vi "Acquisition.vi"(11 "Acq Msg":T2) -> (4 "Display Stream":T1, 5 "Log Stream":T1, 6 "UI Msg":T2)   [LabVIEW 2019, in "Acquisition.lvlib"]
doc: "Message loop for handling messages pertaining to the acquisition of data from the hardware."
uses:
  Acquisition.lvlib
  <extravilib>/ChannelInstances/Messenger-t'Message Queue.lvlib-Message Cluster.ctl'/))Channel.ctl
  support/Message Queue/Message Cluster.ctl
  <extravilib>/ChannelInstances/Stream-var/)Channel.ctl
  HeatFlow/HeatFlow HW Tasks.ctl
  Acquisition State.ctl
  Settings/Settings.ctl
  Settings/Runtime Conf.ctl
  HeatFlow/HeatFlow HW Cfg.ctl
  HeatFlow/HeatFlow Acq Data.ctl
  <extravilib>/ChannelInstances/Stream-var/Write With Abort.vi
  <extravilib>/ChannelInstances/Stream-var/Endpoint.vi
  <extravilib>/ChannelInstances/Messenger-t'Message Queue.lvlib-Message Cluster.ctl'/Instantiate.vi
  <vilib>/Utility/error.llb/Error Cluster From Error Code.vi
  <extravilib>/ChannelInstances/Stream-var/)Channel.vi
  <resource>/ChannelSupport/_ChannelSupport/WaitIfNeeded.vi
  <vilib>/ErrorRing/Error Ring.xnode
  support/Message Queue/Message Queue.lvlib
  Settings/Settings.lvlib
  <extravilib>/ChannelInstances/Stream-var.lvlib
  <extravilib>/ChannelInstances/Messenger-t'Message Queue.lvlib-Message Cluster.ctl'.lvlib
panel:
  in  "Wart zwrotna":dbl
  out "Time":dbl
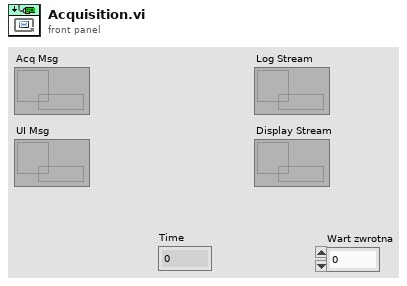
[diagram p1: front panel]
types:
  T1 = typedef "Stream-var.lvlib/)Channel.ctl" = refnum<queue>
  T2 = typedef "Messenger-t'Message Queue.lvlib-Message Cluster.ctl'.lvlib/))Channel.ctl" = refnum<queue>
  T3 = typedef "Acquisition.lvlib/HeatFlow HW Cfg.ctl" = cluster{"Heater Temp":cluster{"On":bool, "Min Val":dbl, "Max Val":dbl, "Units":string}, "LakeShore Temp":cluster{"On":bool, "Min Val":dbl, "Max Val":dbl, "Units":string}, "Heater Ctrl":cluster{"On":bool, "Min Val":dbl, "Max Val":dbl}, "TEG Load dU":cluster{"On":bool, "Min Val":dbl, "Max Val":dbl}, "Heater dU":cluster{"On":bool, "Min Val":dbl, "Max Val":dbl}, "I Res dU":cluster{"On":bool, "Min Val":dbl, "Max Val":dbl}, "Is Conf Set Up":bool}
  T4 = typedef "Settings.lvlib/Settings.ctl" = cluster{"Runtime":T5, "Cfg Files Dir":path, "Cfg File":path}
  T5 = typedef "Settings.lvlib/Runtime Conf.ctl" = cluster{"Time Interval, s":dbl, "Time Resolution, ms":u32, "Hot Side MOS, V":dbl, "Cold Side MOS, V":dbl}
  T6 = typedef "Acquisition.lvlib/Acquisition State.ctl" = enum16{"Idle", "Acquiring"}
  T7 = typedef "Acquisition.lvlib/HeatFlow HW Tasks.ctl" = cluster{"Heater Temp Task":refnum<k21>, "Heater Ctrl Task":refnum<k21>, "TEG Load dU Task":refnum<k21>, "Heater dU Task":refnum<k21>, "I Res dU Task":refnum<k21>, "LakeShore Temp":refnum<visa-resource-name>}
  T8 = typedef "Logging.lvlib/HeatFlow Res Cfg.ctl" = cluster{"Heater Temp":cluster{"On":bool, "Min Val":dbl, "Max Val":dbl, "Units":string}, "Tube Temp":cluster{"On":bool, "Min Val":dbl, "Max Val":dbl, "Units":string}, "Hot Heater Power":cluster{"On":bool, "Min Val":dbl, "Max Val":dbl, "Units":string}, "TEG Power":cluster{"On":bool, "Min Val":dbl, "Max Val":dbl, "Units":string}, "Details":bool, "Heater dU":cluster{"Min Val":dbl, "Max Val":dbl, "Units":string}, "I Res dU":cluster{"Min Val":dbl, "Max Val":dbl, "Units":string}}
  T9 = typedef "Acquisition.lvlib/HeatFlow Acq Data.ctl" = cluster{"Time Stamp":timestamp, "Time Delta":u32, "LakeShore_Temp":cluster{"Tube_T_1":dbl, "Tube_T_2":dbl, "Tube_T_3":dbl, "Tube_T_4":dbl, "Tube_T_5":dbl, "Tube_T_6":dbl, "Tube_T_7":dbl, "Tube_T_8":dbl}, "Heaters":cluster{"I_Res_dU":dbl, "Heater_dU":dbl, "Hot_Side_I":dbl, "Hot_Side_P":dbl, "Cold_Ctrl_U":dbl, "Hot_Ctrl_U":dbl, "Hot_Side_T":dbl, "Cold_Side_T":dbl}, "TEG":cluster{"TEG_Load_dU":dbl, "TEG_Load_R":dbl, "TEG_Load_I":dbl, "TEG_Load_P":dbl, "TEG_eta":dbl, "TEG_dT":dbl, "TEG_U_open":dbl, "TEG_U_Test":dbl, "TEG_R_Test":dbl, "TEG_Rw":dbl}, "LastElement?":bool}
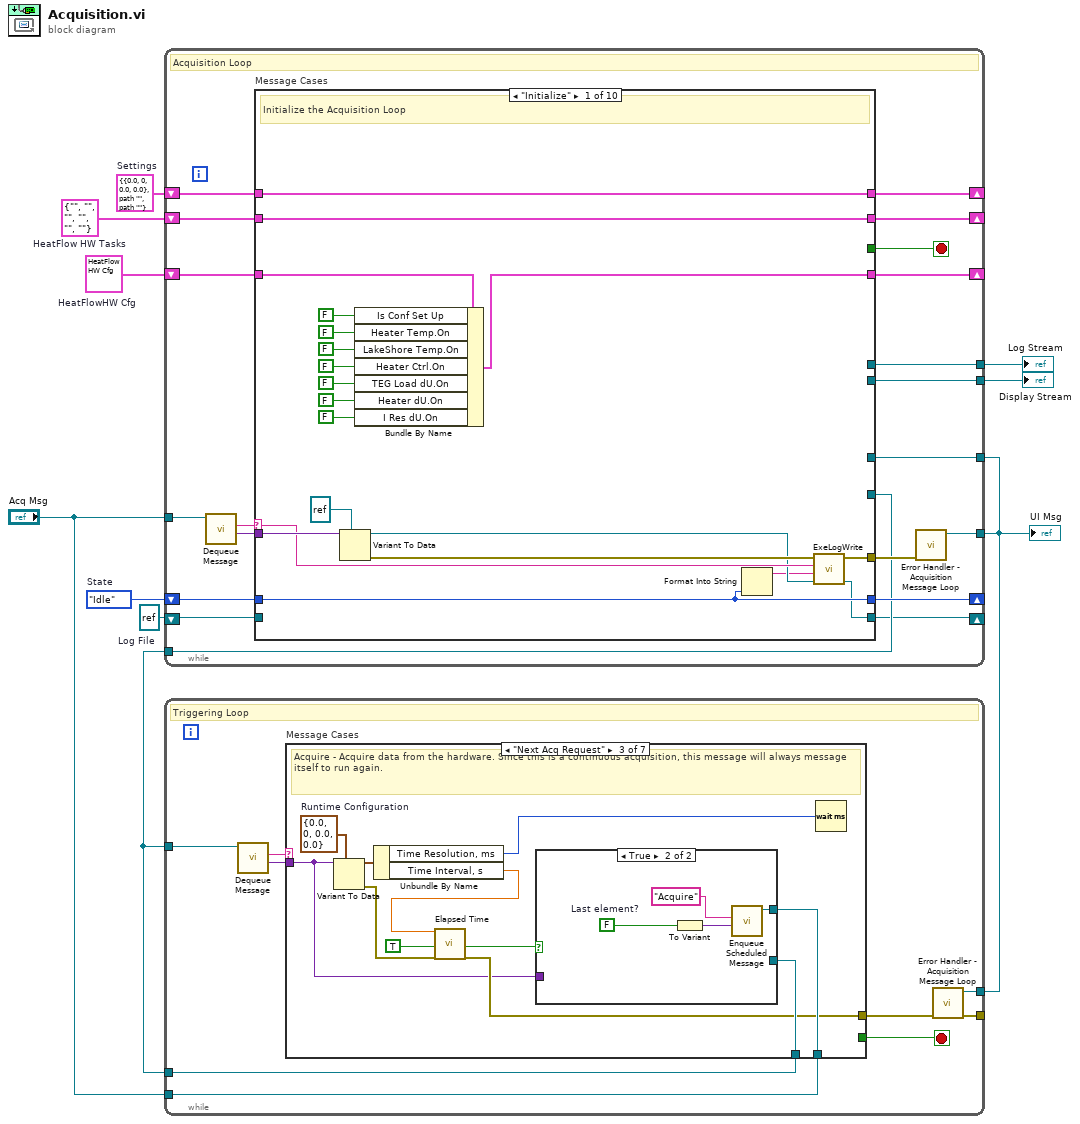
[diagram p0: block diagram]
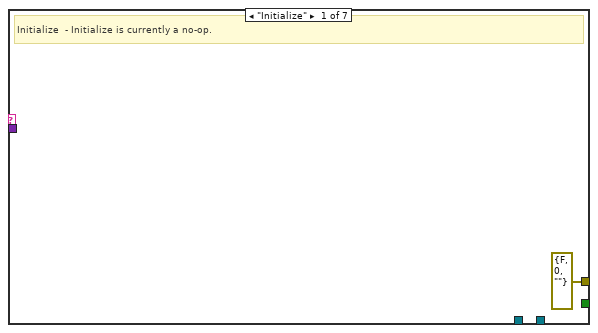
[diagram p2: hidden frame]
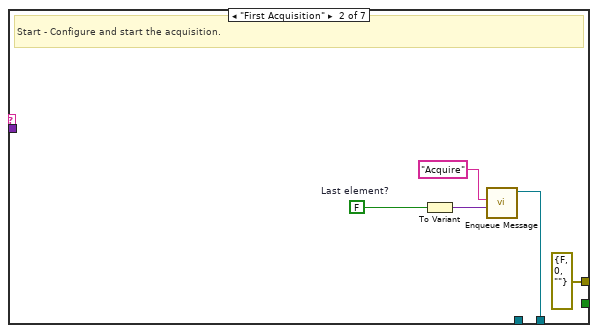
[diagram p3: hidden frame]
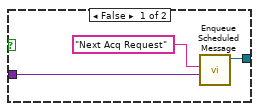
[diagram p4: hidden frame]
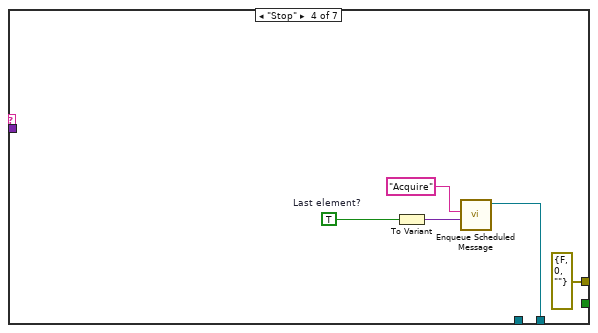
[diagram p5: hidden frame]
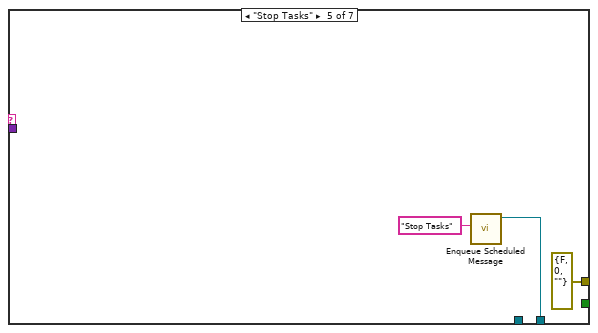
[diagram p6: hidden frame]
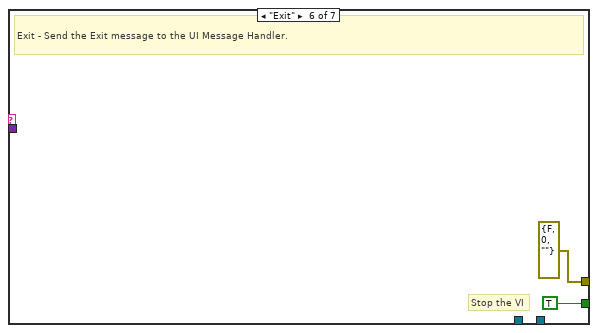
[diagram p7: hidden frame]
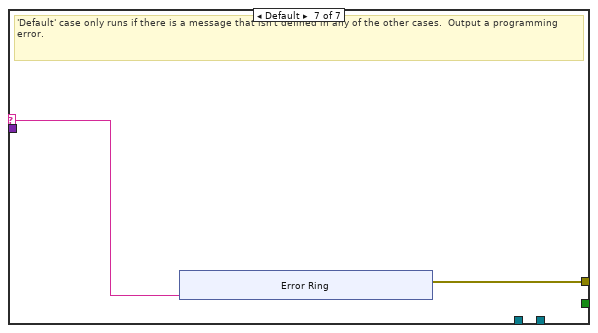
[diagram p8: hidden frame]
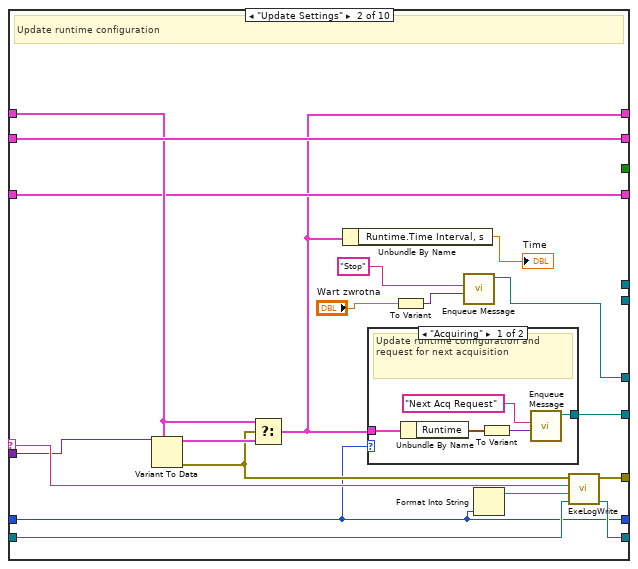
[diagram p9: hidden frame]
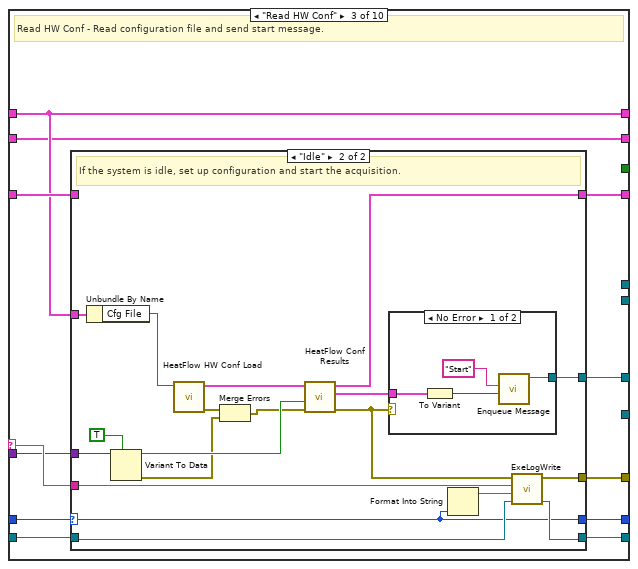
[diagram p11: hidden frame]
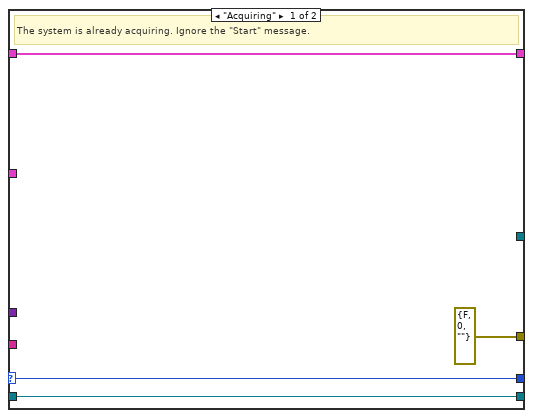
[diagram p12: hidden frame]
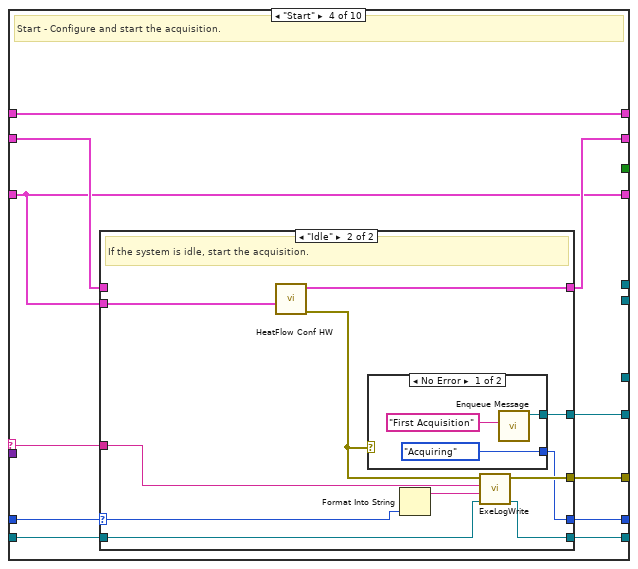
[diagram p14: hidden frame]
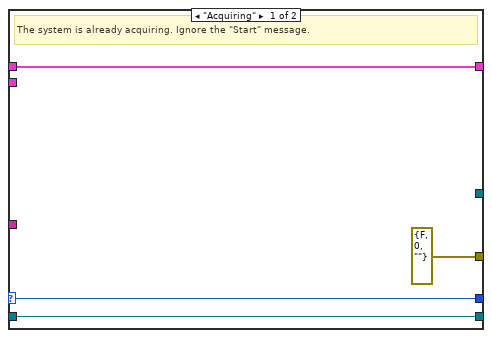
[diagram p15: hidden frame]
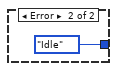
[diagram p16: hidden frame]
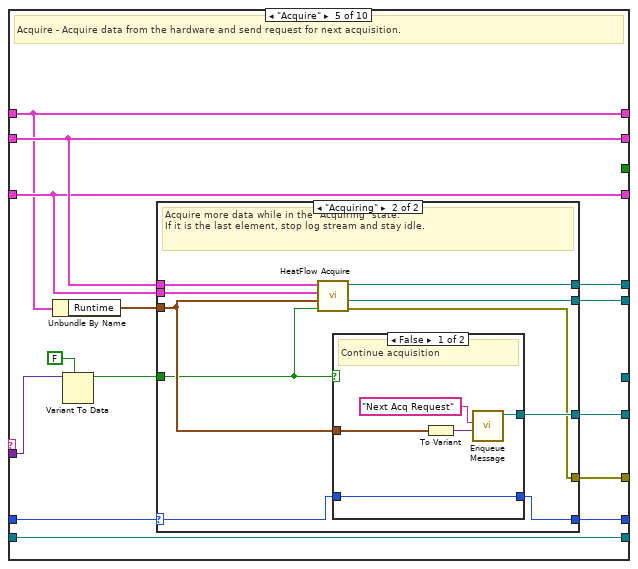
[diagram p17: hidden frame]
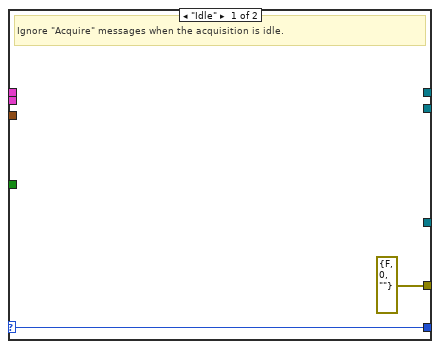
[diagram p18: hidden frame]
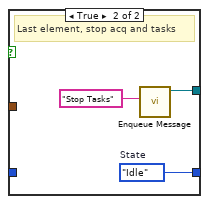
[diagram p19: hidden frame]
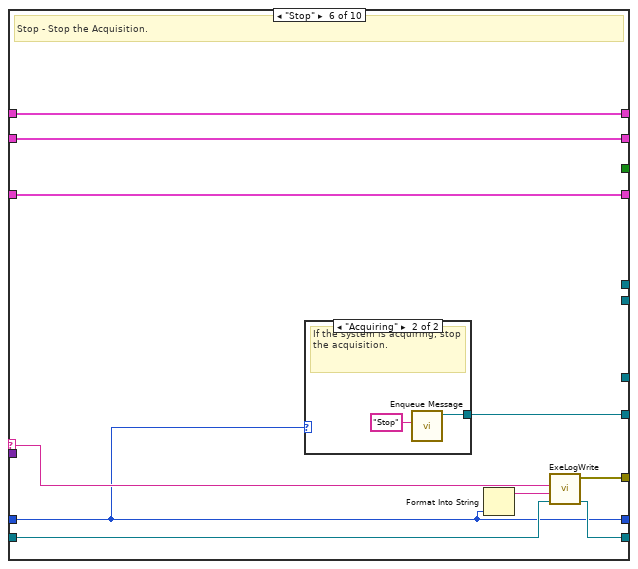
[diagram p20: hidden frame]
diagram:
  w1 = T3 {"Heater Temp"={"On"=FALSE, "Min Val"=0.0, "Max Val"=0.0, "Units"=""}, "LakeShore Temp"={"On"=FALSE, "Min Val"=0.0, "Max Val"=0.0, "Units"=""}, "Heater Ctrl"={"On"=FALSE, "Min Val"=0.0, "Max Val"=0.0}, "TEG Load dU"={"On"=FALSE, "Min Val"=0.0, "Max Val"=0.0}, "Heater dU"={"On"=FALSE, "Min Val"=0.0, "Max Val"=0.0}, "I Res dU"={"On"=FALSE, "Min Val"=0.0, "Max Val"=0.0}, "Is Conf Set Up"=FALSE}  # HeatFlowHW Cfg
  w4 = T4 {"Runtime"={"Time Interval, s"=0.0, "Time Resolution, ms"=0, "Hot Side MOS, V"=0.0, "Cold Side MOS, V"=0.0}, "Cfg Files Dir"=path "", "Cfg File"=path ""}  # Settings
  w5 = refnum<file> refnum  # Log File
  w7 = Acquisition_State."Idle"  # State
  w8 = T7 {"Heater Temp Task"="", "Heater Ctrl Task"="", "TEG Load dU Task"="", "Heater dU Task"="", "I Res dU Task"="", "LakeShore Temp"=""}  # HeatFlow HW Tasks
  n1 = while {
    shift-right: [w29] -> _
    shift-left: w8 -> [w30]
    shift-right: [w27] -> _
    shift-left: w7 -> [w28]
    shift-right: [w25] -> _
    shift-left: w4 -> [w26]
    tunnel: "Acq Msg" -> [w19]
    tunnel: [w21] -> w10
    tunnel: w10 -> [w20]
    tunnel: w6 -> [w18]
    shift-right: [w15] -> _
    shift-left: w5 -> [w16]
    shift-right: [w13] -> _
    shift-left: w1 -> [w14]
    tunnel: [w12] -> w3
    tunnel: [w11] -> w2
    stop <- w17 stop-if-true
    # "Acquisition Loop"
    n2 = call "Dequeue Message.vi"("channel"=w19) -> ("message data"=w23:variant, "message"=w24:string)  [unwired: 8 in, 1 out]
    n3 = case "Message Cases" shown="\"Initialize\"" w24 {
      selector: w24 -> [w45 w66 w81 w118 _ w183 w196 w213 w234 w245]
      tunnel: [w41 w65 w86 w124 w157 w181 w193 w214 w229 w246] -> w22
      tunnel: w30 -> [w50 w62 w76 w116 w152 w180 w192 w212 w241 w248]
      tunnel: [w50 w62 w76 w115 w152 w180 w192 w212 w241 w248] -> w29
      tunnel: w28 -> [w43 w57 w84 w122 w155 w178 w190 w207 w235 w247]
      tunnel: [w43 w57 w85 w123 w156 w178 w190 w207 w235 w247] -> w27
      tunnel: w26 -> [w49 w59 w78 w117 w149 w187 w200 w210 w240 w244]
      tunnel: [w49 w56 w78 w117 w149 w187 w200 w210 w240 w244] -> w25
      tunnel: w23 -> [w47 w63 w75 _ w147 _ _ _ _ _]
      tunnel: [_ w60 _ w121 w154 w186 _ _ w239 _] -> w18
      tunnel: [_ w54 w77 _ _ _ w199 _ _ _] -> w20
      tunnel: [_ _ _ _ _ _ _ _ TRUE _] -> w17
      tunnel: w16 -> [_ w69 w83 w120 w153 w184 w197 w208 w233 w243]
      tunnel: [w40 w68 w82 w119 w153 w182 w195 w208 refnum<file> refnum ("Log File") w243] -> w15
      tunnel: w14 -> [w39 w58 w80 w114 w151 w179 w191 w211 w232 w242]
      tunnel: [w31 w58 w79 w114 w151 w179 w191 w211 w232 w242] -> w13
      tunnel: [_ _ _ _ w145 _ _ _ _ _] -> w12
      tunnel: [_ _ _ _ w144 _ _ _ w224 _] -> w11
      frame "Initialize" {
        # "Initialize the Acquisition Loop"
        n4 = Variant To Data(type=refnum<file> refnum ("refnum out"), Variant=w47) -> (data=w44:refnum<file>, error out=w46:errorcluster)  [unwired: 1 in]
        n5 = Bundle By Name(cluster=w39, "Is Conf Set Up"=FALSE ("HW.Is Conf Set Up"), "Heater Temp.On"=FALSE ("HW.Heater Temp.On"), "LakeShore Temp.On"=FALSE ("HW.LakeShore Temp.On"), "Heater Ctrl.On"=FALSE ("HW.Heater Ctrl.On"), "TEG Load dU.On"=FALSE ("HW.TEG Load dU.On"), "Heater dU.On"=FALSE ("HW.Heater dU.On"), "I Res dU.On"=FALSE ("HW.I Res dU.On")) -> (w31:T3)
        n6 = Format Into String(w43) -> (resulting string=w42:string)  [unwired: 3 in, 1 out]
        n7 = call "ExeLogWrite.vi"("refnum in"=w44, "State"=w42, "Message"=w45, "error in"=w46) -> ("refnum out"=w40:refnum<file>, "error out"=w41:errorcluster)  [unwired: 6 in]
      }
      frame "Update Settings" {
        # "Update runtime configuration"
        n8 = Variant To Data(type=w59, Variant=w63) -> (data=w64:T4, error out=w61:errorcluster)  [unwired: 1 in]
        n9 = Select(t=w59, s=w61, f=w64) -> (s? t:f=w56:T4)
        n10 = Unbundle By Name(w56) -> ("Runtime.Time Interval, s"=→"Time":dbl)
        n11 = case shown="\"Acquiring\"" w57 {
          tunnel: [w74 _] -> w60
          tunnel: w56 -> [w71 _]
          frame "Acquiring" {
            # "Update runtime configuration and request for next acquisition"
            n12 = Unbundle By Name(w71) -> ("Runtime"=w70:T5)
            n13 = To Variant(anything=w70) -> (Variant=w72:variant)
            n14 = call "Enqueue Message.vi"("data (empty)"=w72, "message"="Next Acq Request") -> ("channel"=w74:T2)  [unwired: 9 in]
          }
          frame "Idle" {
            # "Update runtime configuration and stay idle"
          }
        }
        n15 = To Variant(anything="Wart zwrotna") -> (Variant=w51:variant)
        n16 = call "Enqueue Message.vi"("data (empty)"=w51, "message"="Stop") -> ("channel"=w54:T2)  [unwired: 9 in]
        n17 = Format Into String(w57) -> (resulting string=w67:string)  [unwired: 3 in, 1 out]
        n18 = call "ExeLogWrite.vi"("refnum in"=w69, "State"=w67, "Message"=w66, "error in"=w61) -> ("refnum out"=w68:refnum<file>, "error out"=w65:errorcluster)  [unwired: 6 in]
      }
      frame "Read HW Conf" {
        # "Read HW Conf - Read configuration file and send start message."
        n19 = case shown="\"Idle\"" w84 {
          selector: w84 -> [w90 w104]
          tunnel: [errorcluster {"status"=FALSE, "code"=0, "source"=""} ("error IO") w101] -> w86
          tunnel: [w90 w104] -> w85
          tunnel: w83 -> [w89 w107]
          tunnel: [w89 w106] -> w82
          tunnel: w81 -> [_ w108]
          tunnel: w80 -> [w88 _]
          tunnel: [w88 w97] -> w79
          tunnel: w78 -> [_ w103]
          tunnel: [_ w105] -> w77
          tunnel: w75 -> [_ w99]
          frame "Acquiring" {
            # "The system is already acquiring. Ignore the \"Start\" message."
          }
          frame "Idle" {
            # "If the system is idle, set up configuration and start the acquisition."
            n20 = Unbundle By Name(w103) -> ("Cfg File"=w102:path)
            n21 = Variant To Data(type=TRUE, Variant=w99) -> (data=w96:bool, error out=w93:errorcluster)  [unwired: 1 in]
            n22 = call "HeatFlow HW Conf Load.vi"("Conf File"=w102) -> ("error out"=w92:errorcluster, "HeatFlow HW Cfg"=w95:T3)  [unwired: 9 in]
            n23 = Merge Errors(w92, w93) -> (w91:errorcluster)
            n24 = call "HeatFlow Conf Results.vi"("error in"=w91, "All signals?"=w96, "HW Cfg In"=w95) -> ("error out"=w98:errorcluster, "HeatFlowRes Cfg"=w94:T8, "HW Cfg Out"=w97:T3)  [unwired: 6 in]
            n25 = case shown="No Error" w98 {
              tunnel: [w112 _] -> w105
              tunnel: w94 -> [w110 _]
              frame No Error {
                n26 = To Variant(anything=w110) -> (Variant=w111:variant)
                n27 = call "Enqueue Message.vi"("data (empty)"=w111, "message"="Start" ("Message")) -> ("channel"=w112:T2)  [unwired: 9 in]
              }
              frame Error {
              }
            }
            n28 = Format Into String(w104) -> (resulting string=w109:string)  [unwired: 3 in, 1 out]
            n29 = call "ExeLogWrite.vi"("refnum in"=w107, "State"=w109, "Message"=w108, "error in"=w98) -> ("refnum out"=w106:refnum<file>, "error out"=w101:errorcluster)  [unwired: 6 in]
          }
        }
      }
      frame "Start" {
        # "Start - Configure and start the acquisition."
        n30 = case shown="\"Idle\"" w122 {
          selector: w122 -> [w128 w138]
          tunnel: [errorcluster {"status"=FALSE, "code"=0, "source"=""} ("error IO") w132] -> w124
          tunnel: [w128 w131] -> w123
          tunnel: [_ w139] -> w121
          tunnel: w120 -> [w127 w135]
          tunnel: [w127 w134] -> w119
          tunnel: w118 -> [_ w136]
          tunnel: w116 -> [w126 _]
          tunnel: [w126 w133] -> w115
          tunnel: w114 -> [_ w129]
          frame "Acquiring" {
            # "The system is already acquiring. Ignore the \"Start\" message."
          }
          frame "Idle" {
            # "If the system is idle, start the acquisition."
            n31 = call "HeatFlow Conf HW.vi"("HeatFlowHW Cfg"=w129) -> ("error out"=w130:errorcluster, "Hardware Tasks out"=w133:T7)  [unwired: 9 in]
            n32 = case shown="No Error" w130 {
              tunnel: [w141 _] -> w139
              tunnel: [Acquisition_State."Acquiring" ("Acquisition State") Acquisition_State."Idle" ("Acquisition State")] -> w131
              frame No Error {
                n33 = call "Enqueue Message.vi"("message"="First Acquisition" ("Message")) -> ("channel"=w141:T2)  [unwired: 10 in]
              }
              frame Error {
              }
            }
            n34 = Format Into String(w138) -> (resulting string=w137:string)  [unwired: 3 in, 1 out]
            n35 = call "ExeLogWrite.vi"("refnum in"=w135, "State"=w137, "Message"=w136, "error in"=w130) -> ("refnum out"=w134:refnum<file>, "error out"=w132:errorcluster)  [unwired: 6 in]
          }
        }
      }
      frame "Acquire" {
        # "Acquire - Acquire data from the hardware and send request for next acquisition."
        n36 = Unbundle By Name(w149) -> ("Runtime"=w150:T5)
        n37 = Variant To Data(type=FALSE, Variant=w147) -> (data=w148:bool)  [unwired: 1 in, 1 out]
        n38 = case shown="\"Acquiring\"" w155 {
          selector: w155 -> [w159 w163]
          tunnel: [errorcluster {"status"=FALSE, "code"=0, "source"=""} ("error IO") w166] -> w157
          tunnel: w152 -> [_ w168]
          tunnel: [w159 w164] -> w156
          tunnel: [_ w169] -> w154
          tunnel: w151 -> [_ w167]
          tunnel: w150 -> [_ w165]
          tunnel: w148 -> [_ w162]
          tunnel: [_ w161] -> w145
          tunnel: [_ w160] -> w144
          frame "Idle" {
            # "Ignore \"Acquire\" messages when the acquisition is idle."
          }
          frame "Acquiring" {
            # "Acquire more data while in the \"Acquiring\" state.\nIf it is the last element, stop log stream and stay idle."
            n39 = call "HeatFlow Acquire.vi"("HeatFlow HW Tasks in"=w168, "HeatFlow HW Cfg"=w167, "Runtime"=w165, "Last element?"=w162) -> ("Log Stream"=w161:T1, "Display Stream"=w160:T1, "error out"=w166:errorcluster)  [unwired: 4 in]
            n40 = case shown="False" w162 {
              tunnel: [w174 w176] -> w169
              tunnel: w165 -> [w171 _]
              tunnel: [w170 w177] -> w164
              tunnel: w163 -> [w170 _]
              frame False {
                # "Continue acquisition"
                n41 = To Variant(anything=w171) -> (Variant=w172:variant)
                n42 = call "Enqueue Message.vi"("data (empty)"=w172, "message"="Next Acq Request") -> ("channel"=w174:T2)  [unwired: 9 in]
              }
              frame True {
                w177 = Acquisition_State."Idle"  # State
                # "Last element, stop acq and tasks"
                n43 = call "Enqueue Message.vi"("message"="Stop Tasks") -> ("channel"=w176:T2)  [unwired: 10 in]
              }
            }
          }
        }
      }
      frame "Stop" {
        # "Stop - Stop the Acquisition."
        n44 = case shown="\"Acquiring\"" w178 {
          tunnel: [_ w189] -> w186
          frame "Idle" {
            # "The system is already idle. Ignore the \"Stop\" message."
          }
          frame "Acquiring" {
            # "If the system is acquiring, stop the acquisition."
            n45 = call "Enqueue Message.vi"("message"="Stop") -> ("channel"=w189:T2)  [unwired: 10 in]
          }
        }
        n46 = Format Into String(w178) -> (resulting string=w185:string)  [unwired: 3 in, 1 out]
        n47 = call "ExeLogWrite.vi"("refnum in"=w184, "State"=w185, "Message"=w183) -> ("refnum out"=w182:refnum<file>, "error out"=w181:errorcluster)  [unwired: 7 in]
      }
      frame "Stop Tasks" {
        # "Stop - Stop the Acquisition."
        n48 = case shown="\"Idle\"" w190 {
          tunnel: [w201 errorcluster {"status"=FALSE, "code"=0, "source"=""} ("error out")] -> w194
          tunnel: [w204 _] -> w199
          tunnel: w192 -> [w203 _]
          tunnel: w191 -> [w202 _]
          frame "Idle" {
            # "If the system is idle, stop all tasks."
            n49 = call "HeatFlow Stop Acq Tasks.vi"("HeatFlow HW Cfg"=w202, "HeatFlow HW Tasks in"=w203) -> ("error out"=w201:errorcluster)  [unwired: 9 in]
            n50 = call "Enqueue Message.vi"("message"="Acquisition Stopped") -> ("channel"=w204:T2)  [unwired: 10 in]
          }
          frame "Acquiring" {
            # "Don't stop tasks while system is aquiring."
          }
        }
        n51 = Format Into String(w190) -> (resulting string=w198:string)  [unwired: 3 in, 1 out]
        n52 = call "ExeLogWrite.vi"("refnum in"=w197, "State"=w198, "Message"=w196, "error in"=w194) -> ("refnum out"=w195:refnum<file>, "error out"=w193:errorcluster)  [unwired: 6 in]
      }
      frame "Save HW Conf" {
        # "Read HW Conf - Read configuration file and send start message."
        n53 = Unbundle By Name(w210) -> ("Cfg File"=w209:path)
        n54 = case shown="\"Idle\"" w207 {
          selector: w207 -> [_ w221]
          tunnel: [errorcluster {"status"=FALSE, "code"=0, "source"=""} ("error out") w219] -> w214
          tunnel: w213 -> [_ w222]
          tunnel: w211 -> [_ w218]
          tunnel: w209 -> [_ w217]
          tunnel: w208 -> [_ w216]
          frame "Acquiring" {
            # "The system is already acquiring. Ignore the \"Save\" message."
          }
          frame "Idle" {
            # "If the system is idle, save configuration file."
            n55 = Format Into String(w221) -> (resulting string=w223:string)  [unwired: 3 in, 1 out]
            n56 = call "HeatFlow HW Conf Save.vi"("HeatFlow HW Cfg"=w218, "Conf File"=w217) -> ("error out"=w220:errorcluster)  [unwired: 8 in]
            n57 = call "ExeLogWrite.vi"("refnum in"=w216, "State"=w223, "Message"=w222, "error in"=w220) -> ("error out"=w219:errorcluster)  [unwired: 6 in, 1 out]
          }
        }
      }
      frame "Exit" {
        w227 = T9 {"Time Stamp"=timestamp(0 s since 1904-01-01), "Time Delta"=0, "LakeShore_Temp"={"Tube_T_1"=0.0, "Tube_T_2"=0.0, "Tube_T_3"=0.0, "Tube_T_4"=0.0, "Tube_T_5"=0.0, "Tube_T_6"=0.0, "Tube_T_7"=0.0, "Tube_T_8"=0.0}, "Heaters"={"I_Res_dU"=0.0, "Heater_dU"=0.0, "Hot_Side_I"=0.0, "Hot_Side_P"=0.0, "Cold_Ctrl_U"=0.0, "Hot_Ctrl_U"=0.0, "Hot_Side_T"=0.0, "Cold_Side_T"=0.0}, "TEG"={"TEG_Load_dU"=0.0, "TEG_Load_R"=0.0, "TEG_Load_I"=0.0, "TEG_Load_P"=0.0, "TEG_eta"=0.0, "TEG_dT"=0.0, "TEG_U_open"=0.0, "TEG_U_Test"=0.0, "TEG_R_Test"=0.0, "TEG_Rw"=0.0}, "LastElement?"=FALSE}  # HeatFlow Acq Data
        w225 = TRUE  # last element?
        # "Send Abort to Display Loop"
        # "Stop the VI"
        # "Exit - Send the Exit message to the UI Message Handler."
        n58 = Format Into String(w235) -> (resulting string=w236:string)  [unwired: 3 in, 1 out]
        n59 = call "ExeLogWrite.vi"("refnum in"=w233, "State"=w236, "Message"=w234) -> ("refnum out"=w230:refnum<file>, "error out"=w231:errorcluster)  [unwired: 7 in]
        n60 = Close File(refnum=w230, error in=w231) -> (error out=w229:errorcluster)  [unwired: 1 out]
        n61 = To Variant(anything=w227) -> (Variant=w226:variant)
        n62 = call <extravilib>:"Write.vi"("last element? (F)"=w225, "element"=w226) -> ("channel"=w224:T1)  [unwired: 7 in, 2 out]
        n63 = call "Enqueue Message.vi"("message"="Exit") -> ("channel"=w239:T2)  [unwired: 10 in]
      }
      frame Default {
        # "'Default' case only runs if there is a message that isn't defined in any of the other cases."
        n64 = xnode "Error Ring"("parameter 0"=w245) -> ("error out"=w246:errorcluster)
      }
    }
    n65 = call "Error Handler - Acquisition Message Loop.vi"("error in (no error)"=w22) -> ("UI Channel"=w21:T2)  [unwired: 9 in, 1 out]
  }
  "UI Msg" <- w10
  "Log Stream" <- w3
  "Display Stream" <- w2
  n66 = while {
    tunnel: [w261] -> _
    tunnel: w6 -> [w259]
    tunnel: w10 -> [w260]
    tunnel: "Acq Msg" -> [w257]
    tunnel: [w258] -> w6
    stop <- w256 stop-if-true
    # "Triggering Loop"
    n67 = call "Dequeue Message.vi"("channel"=w259) -> ("message data"=w263:variant, "message"=w264:string)  [unwired: 8 in, 1 out]
    n68 = case "Message Cases" shown="\"Next Acq Request\"" w264 {
      selector: w264 -> [_ _ _ _ _ _ w299]
      tunnel: [errorcluster {"status"=FALSE, "code"=0, "source"=""} ("error out") errorcluster {"status"=FALSE, "code"=0, "source"=""} ("error out") w272 errorcluster {"status"=FALSE, "code"=0, "source"=""} ("error out") errorcluster {"status"=FALSE, "code"=0, "source"=""} ("error out") errorcluster {"status"=FALSE, "code"=0, "source"=""} ("error out") w300] -> w262
      tunnel: [_ _ _ _ _ TRUE _] -> w256
      tunnel: w263 -> [_ _ w271 _ _ _ _]
      tunnel: [_ _ w274 _ _ _ _] -> w258
      tunnel: [_ w269 w273 w291 w295 _ _] -> w257
      frame "Initialize" {
        # "Initialize  - Initialize is currently a no-op."
      }
      frame "First Acquisition" {
        w267 = FALSE  # Last element?
        # "Start - Configure and start the acquisition."
        n69 = To Variant(anything=w267) -> (Variant=w266:variant)
        n70 = call "Enqueue Message.vi"("data (empty)"=w266, "message"="Acquire") -> ("channel"=w269:T2)  [unwired: 9 in]
      }
      frame "Next Acq Request" {
        w281 = T5 {"Time Interval, s"=0.0, "Time Resolution, ms"=0, "Hot Side MOS, V"=0.0, "Cold Side MOS, V"=0.0}  # Runtime Configuration
        # "Acquire - Acquire data from the hardware. Since this is a continuous acquisition, this message will always message itself to run again."
        n71 = Variant To Data(type=w281, Variant=w271) -> (data=w280:T5, error out=w276:errorcluster)  [unwired: 1 in]
        n72 = Unbundle By Name(w280) -> ("Time Resolution, ms"=w279:u32, "Time Interval, s"=w278:dbl)
        n73 = call "Elapsed Time"("Time Target (s)"=w278, "Auto Reset"=TRUE, "error in (no error)"=w276) -> ("Time has Elapsed"=w275:bool, "error out"=w272:errorcluster)  [unwired: 9 in, 6 out]
        n74 = case shown="True" w275 {
          tunnel: [_ w287] -> w273
          tunnel: [w283 _] -> w274
          tunnel: w271 -> [w282 _]
          frame False {
            n75 = call "Enqueue Scheduled Message.vi"("data (empty)"=w282, "message"="Next Acq Request") -> ("channel"=w283:T2)  [unwired: 8 in, 1 out]
          }
          frame True {
            w285 = FALSE  # Last element?
            n76 = To Variant(anything=w285) -> (Variant=w286:variant)
            n77 = call "Enqueue Scheduled Message.vi"("data (empty)"=w286, "message"="Acquire" ("Message")) -> ("channel"=w287:T2)  [unwired: 8 in, 1 out]
          }
        }
        n78 = Wait (ms)(milliseconds to wait=w279) -> ()  [unwired: 1 out]
      }
      frame "Stop" {
        w289 = TRUE  # Last element?
        n79 = To Variant(anything=w289) -> (Variant=w290:variant)
        n80 = call "Enqueue Scheduled Message.vi"("data (empty)"=w290, "message"="Acquire") -> ("channel"=w291:T2)  [unwired: 8 in, 1 out]
      }
      frame "Stop Tasks" {
        n81 = call "Enqueue Scheduled Message.vi"("message"="Stop Tasks") -> ("channel"=w295:T2)  [unwired: 9 in, 1 out]
      }
      frame "Exit" {
        # "Stop the VI"
        # "Exit - Send the Exit message to the UI Message Handler."
      }
      frame Default {
        # "'Default' case only runs if there is a message that isn't defined in any of the other cases.  Output a programming error."
        n82 = xnode "Error Ring"("parameter 0"=w299) -> ("error out"=w300:errorcluster)
      }
    }
    n83 = call "Error Handler - Acquisition Message Loop.vi"("error in (no error)"=w262) -> ("dup error in"=w261:errorcluster, "UI Channel"=w260:T2)  [unwired: 9 in]
  }
